vi "TIO RPC Send REQuest.vi"(8 "error in (no error)":errorcluster, 9 "Payload":string, 10 "Topic":string, 11 "TC Connection":T1={"Type"=enum."Serial", "URL"="serial:///dev/cu.usbserial-00000", "TO"=500, "Addr"=0, "Port"=0, "TCP"=refnum, "UDP"=refnum, "Route"=""}) -> (0 "error out":errorcluster, 2 "Request ID":u16=60741 format="%04x", 3 "TC Connection":T1={"Type"=enum."Serial", "URL"="serial:///dev/cu.usbserial-00000", "TO"=500, "Addr"=0, "Port"=0, "TCP"=refnum, "UDP"=refnum, "Route"=""})   [LabVIEW 2010]
uses:
  <userlib>/TIO Library 2010/TIO SLIP Serial Write.vi
  <userlib>/TIO Library 2010/TIO Form Packet.vi
  <userlib>/TIO Library 2010/TIO SLIP Encode.vi
  <userlib>/TIO Library 2010/TIO Serial Checksum CRC32.vi
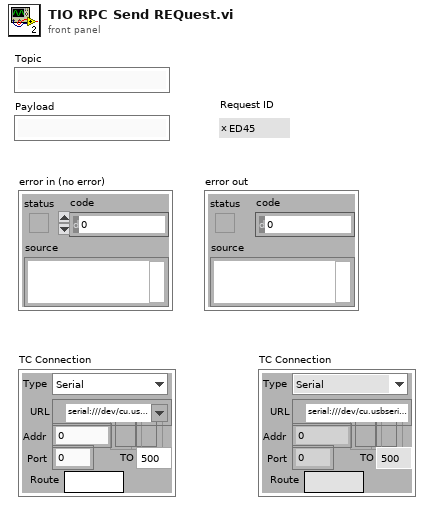
[diagram p1: front panel]
types:
  T1 = cluster{"Type":enum16{"Serial", "TCP", "UDP", "mUDP"}, "URL":refnum<visa-resource-name>, "TO":u32, "Addr":u32, "Port":i32, "TCP":refnum<k5>, "UDP":refnum<k16>, "Route":string}
  T2 = enum8{"Invalid", "Log", "RPC Request", "RPC Reply", "RPC Error", "Stream Description", "User"}
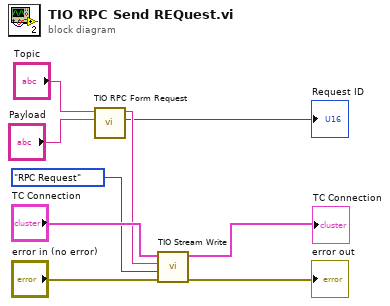
[diagram p0: block diagram]
diagram:
  n1 = call <userlib>:"TIO RPC Form Request.vi"("Payload"="Payload", "Topic"="Topic") -> ("Request ID"=→"Request ID":u16, "String out"=w3:string)  [unwired: 8 in]
  n2 = call <userlib>:"TIO Stream Write.vi"("error in (no error)"="error in (no error)", "Type"=T2."RPC Request", "Payload"=w3, "TC Connection"="TC Connection") -> ("error out"=→"error out":errorcluster, "TC Connection"=→"TC Connection":T1)  [unwired: 5 in]
